vi "setChopFreq.vi"(5 "arrayIn":T1, 7 "startup?":bool=TRUE, 8 "error in (no error)":errorcluster, 9 "emptyVISA":refnum<visa-resource-name>, 10 "newfreq":i32, 11 "VISA resource name":refnum<visa-resource-name>) -> (0 "error out":errorcluster, 1 "Success?":bool=TRUE, 3 "VISA resource name out":refnum<visa-resource-name>)   [LabVIEW 2017, in "LIAinteraction.lvlib"]
uses:
  LIAinteraction.lvlib
  RefArray/RefArray.ctl
  <vilib>/Utility/error.llb/Error Cluster From Error Code.vi
  <vilib>/ErrorRing/Error Ring.xnode
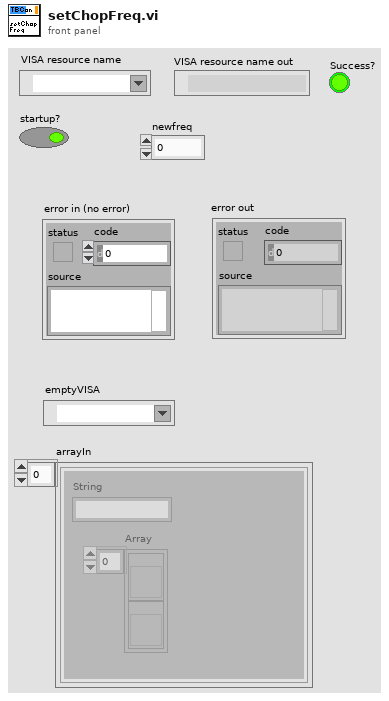
[diagram p1: front panel]
types:
  T1 = typedef "RefArray.ctl" = cluster{"String":string, "Array":refnum<vi>[]}[]
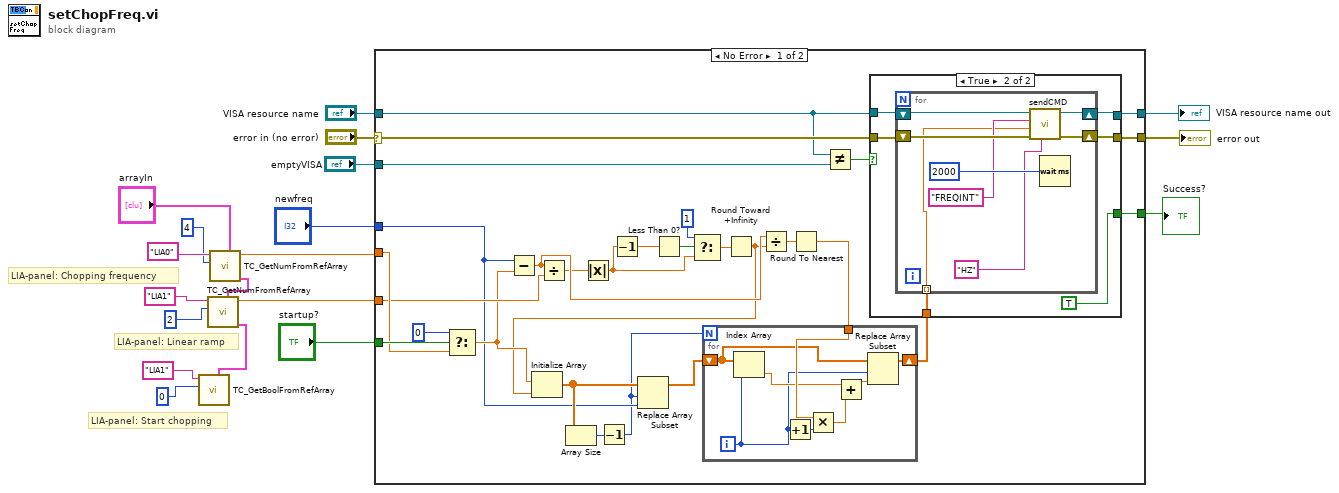
[diagram p0: block diagram]
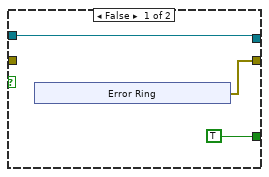
[diagram p2: hidden frame]
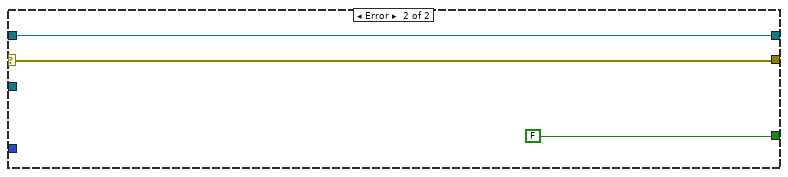
[diagram p3: hidden frame]
diagram:
  # "LIA-panel: Start chopping"
  # "LIA-panel: Chopping frequency"
  # "LIA-panel: Linear ramp"
  n1 = call "TC_GetNumFromRefArray.vi"("arrayIn"="arrayIn", "index"=4, "NameToFind"="LIA0") -> ("arrayOut"=w12:T1, "value"=w1:dbl)  [unwired: 7 in]
  n2 = call "TC_GetNumFromRefArray.vi"("arrayIn"=w12, "index"=2, "NameToFind"="LIA1") -> ("arrayOut"=w8:T1, "value"=w2:dbl)  [unwired: 7 in]
  n3 = call "TC_GetBoolFromRefArray.vi"("arrayIn"=w8, "index"=0, "NameToFind"="LIA1") -> ()  [unwired: 7 in, 2 out]
  n4 = case shown="No Error" "error in (no error)" {
    selector: "error in (no error)" -> [w47 w80]
    tunnel: [w45 w79] -> w19
    tunnel: "VISA resource name" -> [w44 w79]
    tunnel: [w46 w80] -> w17
    tunnel: "newfreq" -> [w26 _]
    tunnel: "emptyVISA" -> [w43 _]
    tunnel: w1 -> [w39 _]
    tunnel: [w41 FALSE] -> w14
    tunnel: "startup?" -> [w40 _]
    tunnel: w2 -> [w33 _]
    frame No Error {
      n5 = Select(t=0, s=w40, f=w39) -> (s? t:f=w29:dbl)
      n6 = Subtract(x=w26, y=w29) -> (x-y=w32:dbl)
      n7 = Divide(x=w32, y=w33) -> (x/y=w31:dbl)
      n8 = Absolute Value(x=w31) -> (abs(x)=w30:dbl)
      n9 = Decrement(x=w30) -> (x-1=w37:dbl)
      n10 = Less Than 0?(x=w37) -> (x < 0?=w36:bool)
      n11 = Select(t=1, s=w36, f=w30) -> (s? t:f=w34:dbl)
      n12 = Round Toward +Infinity(x=w34) -> (ceil(x): smallest int >= x=w21:dbl)
      n13 = Initialize Array(w29, w21) -> (w28:dbl[])
      n14 = Array Size(array=w28) -> (size(s)=w27:i32)
      n15 = Decrement(x=w27) -> (x-1=w20:i32)
      n16 = Replace Array Subset(array=w28, new element=w26, index=w20) -> (w23:dbl[])
      n17 = Divide(x=w32, y=w21) -> (x/y=w25:dbl)
      n18 = Round To Nearest(number=w25) -> (nearest integer value=w24:dbl)
      n19 = for {
        N: w20 -> [_]
        tunnel: w24 -> [w55]
        shift-right: [w50] -> w22
        shift-left: w23 -> [w51]
        i -> [w48]
        n20 = Index Array(array=w51, index=w48) -> (element=w52:dbl)
        n21 = Increment(x=w48) -> (x+1=w49:i32)
        n22 = Multiply(x=w55, y=w49) -> (x*y=w54:dbl)
        n23 = Add(x=w52, y=w54) -> (x+y=w53:dbl)
        n24 = Replace Array Subset(array=w51, new element=w53, index=w48) -> (w50:dbl[])
      }
      n25 = Not Equal?(x=w44, y=w43) -> (x != y?=w42:bool)
      n26 = case shown="True" w42 {
        tunnel: w47 -> [_ w66]
        tunnel: [w56 w67] -> w46
        tunnel: [w58 w68] -> w45
        tunnel: w44 -> [w58 w69]
        tunnel: [TRUE TRUE] -> w41
        tunnel: w22 -> [_ w65]
        frame False {
          n27 = xnode "Error Ring"() -> ("error out"=w56:errorcluster)
        }
        frame True {
          n28 = for {
            shift-right: [w76] -> w68
            shift-left: w69 -> [w77]
            shift-right: [w75] -> w67
            shift-left: w66 -> [w74]
            tunnel: w65 -> [w71] mode=indexing
            n29 = call "sendCMD.vi"("Unit"="HZ", "error in (no error)"=w74, "Value"=w71, "Command"="FREQINT", "VISA resource name"=w77) -> ("error out"=w75:errorcluster, "VISA resource name out"=w76:refnum<visa-resource-name>)  [unwired: 4 in, 1 out]
            n30 = Wait (ms)(milliseconds to wait=2000) -> ()  [unwired: 1 out]
          }
        }
      }
    }
    frame Error {
    }
  }
  "VISA resource name out" <- w19
  "error out" <- w17
  "Success?" <- w14
